vi "DeviceList.vi"(0 "GenericDevice in":refnum<class "GenericDevice.lvclass">, 1 "Delay between send and receive [ms]":i32=5000, 5 "error in (no error)":errorcluster) -> (14 "GenericDevice out":refnum<class "GenericDevice.lvclass">, 15 "results-JSON string":string, 16 "ID":i32, 17 "returned command":string, 18 "error string (if existing)":string, 19 "error out":errorcluster)   [LabVIEW 2023, in "GenericDevice.lvclass"]
uses:
  GenericDevice.lvclass
  GenericDevice.lvclass/GenericDevice.ctl
  eb0e655d-10c0-4d99-92ce-9fce6541daae.vi
  8a7c4e0e-ce51-426b-a457-0e0b7bf85c27.vi
  <vilib>/JDP Science/JSONtext/Variant to JSON Text.vi
  <vilib>/JDP Science/JSONtext/Set Item.vi
  <vilib>/JDP Science/JSONtext/LVClass Serializer/JSONtext LVClass Serializer.lvclass
panel:
  # "Connector Pane"
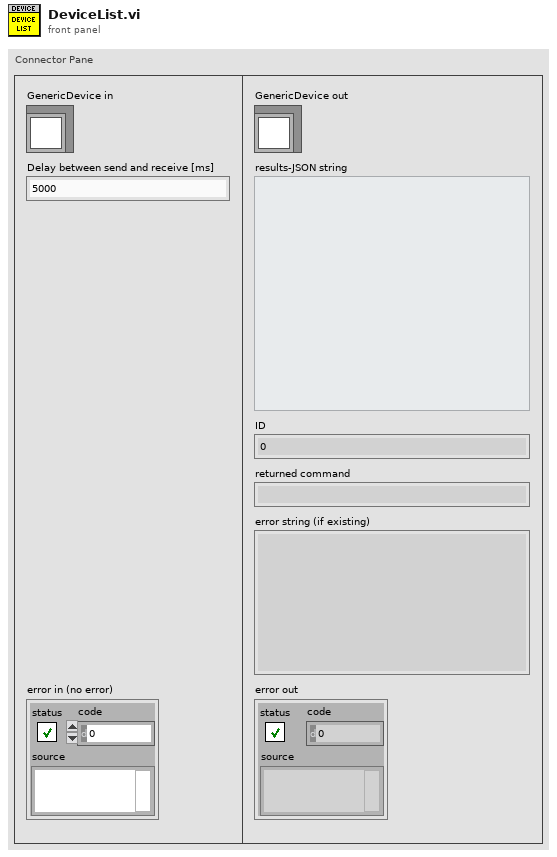
[diagram p1: front panel]
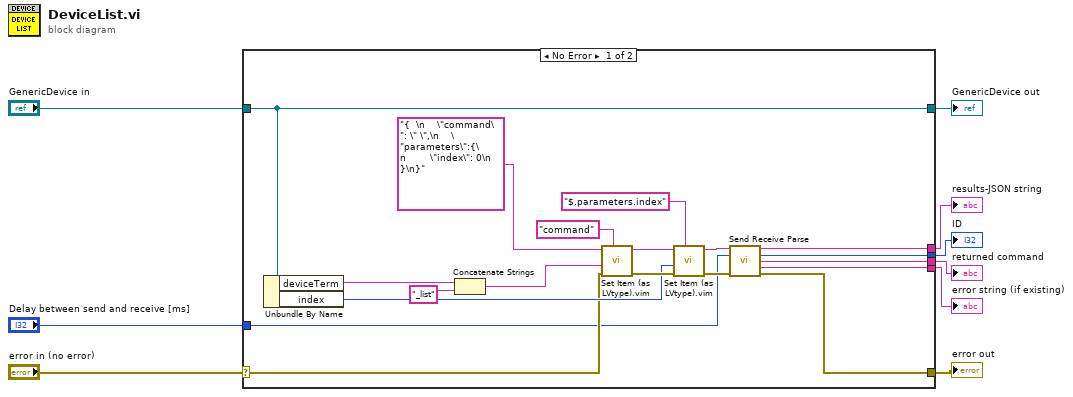
[diagram p0: block diagram]
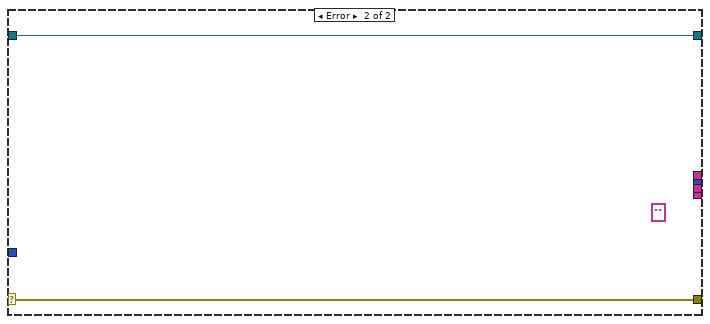
[diagram p2: hidden frame]
diagram:
  n1 = case shown="No Error" "error in (no error)" {
    selector: "error in (no error)" -> [w19 w30]
    tunnel: [w12 w30] -> w8
    tunnel: [w13 w29] -> w6
    tunnel: "GenericDevice in" -> [w13 w29]
    tunnel: [w16 _] -> w5
    tunnel: [w15 _] -> w3
    tunnel: [w14 _] -> w4
    tunnel: [w11 _] -> w2
    tunnel: "Delay between send and receive [ms]" -> [w10 _]
    frame No Error {
      n2 = Unbundle By Name(w13) -> ("deviceTerm"=w24:string, "index"=w20:i32)
      n3 = Concatenate Strings(w24, "_list" ("string")) -> (w21:string)
      n4 = call "Set Item (as LVtype).vim"("$Path or Item Name"="command", "error in (no error)"=w19, "Anything"=w21, "JSON"="{  \n    \"command\": \" \",\n    \"parameters\":{\n        \"index\": 0\n    }\n}") -> ("error out"=w26:errorcluster, "<JSON>"=w27:string)  [unwired: 4 in, 1 out]
      n5 = call "Set Item (as LVtype).vim"("$Path or Item Name"="$.parameters.index", "error in (no error)"=w26, "Anything"=w20, "JSON"=w27) -> ("error out"=w17:errorcluster, "<JSON>"=w18:string)  [unwired: 4 in, 1 out]
      n6 = call "Send Receive Parse.vi"("<JSON>"=w18, "Delay between send and receive [ms]"=w10, "error in"=w17) -> ("results-JSON string"=w11:string, "ID"=w16:i32, "returned command"=w14:string, "error string (if existing)"=w15:string, "error out"=w12:errorcluster)  [unwired: 8 in]
    }
    frame Error {
      (unwired) "" ("<JSON>")
    }
  }
  "error out" <- w8
  "GenericDevice out" <- w6
  "ID" <- w5
  "returned command" <- w4
  "error string (if existing)" <- w3
  "results-JSON string" <- w2
